vi "Array of Variants to JSON Object.vi"(5 "enable LabVIEW extensions? (T)":bool=TRUE, 6 "Pretty Print?":bool, 9 "error in (no error)":errorcluster, 10 "Names":string[](array[string]), 11 "Array":variant[](array[variant])) -> (1 "error out":errorcluster, 3 "<JSON>":string caption="<JSON>Object")   [LabVIEW 2021, in "json.facade.lvlib"]
doc: "Flatten an Array of Variants into a JSON Object. If item names are not supplied, they will be taken from the data name in the Variants.\n\nStrings or Arrays of strings marked with a leading <JSON> tag in their name (including inside clusters) are treated as already being valid JSON. Strings not marked as <JSON> are quoted and escaped as a JSON String."
uses:
  json.facade.lvlib
  jsontext/JSONtext.lvlib
  jsontext/LVClass Serializer/JSONtext LVClass Serializer.lvclass
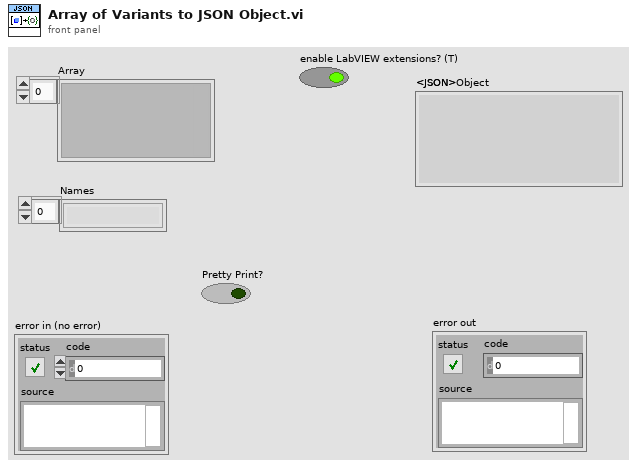
[diagram p1: front panel]
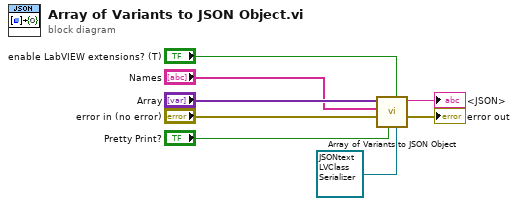
[diagram p0: block diagram]
diagram:
  n1 = call "Array of Variants to JSON Object.vi"("LVClass Serializer"=refnum<class "JSONtext LVClass Serializer.lvclass"> refnum, "enable LabVIEW extensions? (T)"="enable LabVIEW extensions? (T)", "Pretty Print?"="Pretty Print?", "error in (no error)"="error in (no error)", "Names"="Names", "Array"="Array") -> ("error out"=→"error out":errorcluster, "<JSON>"=→"<JSON>":string)  [unwired: 4 in]
